vi "Untitled 2 (SubVI).vi"(10 "Numeric":dbl, 11 "Digital in":refnum<vi>) -> (3 "saturacion":dbl)   [LabVIEW 2018]
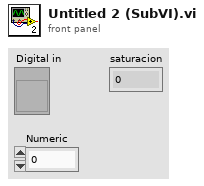
[diagram p1: front panel]
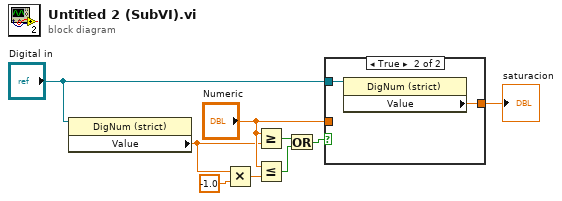
[diagram p0: block diagram]
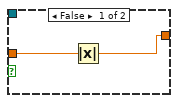
[diagram p2: hidden frame]
diagram:
  n1 = property class="DigNum (strict)"(reference="Digital in") -> ("Value"=w6:dbl)  [unwired: 1 in, 2 out]
  n2 = Multiply(x=w6, y=-1.0) -> (x*y=w4:dbl)
  n3 = Greater Or Equal?(x="Numeric", y=w6) -> (x >= y?=w2:bool)
  n4 = Less Or Equal?(x="Numeric", y=w4) -> (x <= y?=w3:bool)
  n5 = Or(x=w2, y=w3) -> (x .or. y?=w7:bool)
  n6 = case shown="True" w7 {
    tunnel: [w11 w13] -> w8
    tunnel: "Numeric" -> [w10 _]
    tunnel: "Digital in" -> [_ w12]
    frame False {
      n7 = Absolute Value(x=w10) -> (abs(x)=w11:dbl)
    }
    frame True {
      n8 = property class="DigNum (strict)"(reference=w12) -> ("Value"=w13:dbl)  [unwired: 1 in, 2 out]
    }
  }
  "saturacion" <- w8
